vi "FPGA.vi"() -> ()   [LabVIEW 2013]
uses:
  <vilib>/Platform/TimedLoop/XDataNode/timing_clust.ctl
  <vilib>/Platform/TimedLoop/XDataNode/nitl_modes.ctl
  <vilib>/Platform/TimedLoop/XDataNode/wakeup.ctl
  <vilib>/rvi/FXPMathLib/basic elements/FxpIntAccumulator/subVIs/nifxpmath_IntAccumulator_SimConfig.ctl
  <vilib>/rvi/Emulation/niFpgaSctlEmulationGetInTimedLoop.vi
  <vilib>/rvi/Emulation/niFpgaEmulationReportErrorSimple.vi
  <vilib>/rvi/Emulation/niFpgaGetClockAttributes.vi
  <vilib>/rvi/eio/common/nirviEmuTemplateMethod_errors.vi
  <vilib>/rvi/Emulation/niFpgaCriticalErrorInLSC.vi
  <vilib>/rvi/Emulation/niFpgaProcessEmulError.vi
  <vilib>/rvi/Analysis/common/codeGenErrors/XNode/niFpgaXNodeCodeGenErrorHandle.vi
  <vilib>/rvi/FXPMathLib/basic elements/FxpIntAccumulator/simVIs/DllFxpIntAccumulator_sub.vi
  <vilib>/eio/EIONode/EIONode.xnode
  <vilib>/LabVIEW Targets/FPGA/RIO/nicrio_985x_controls.llb/CAN_IO_Frame Cluster.ctl
  <vilib>/LabVIEW Targets/FPGA/RIO/nicrio_985x_controls.llb/CAN_IO_Frame Type.ctl
  <vilib>/rvi/Analysis/measure/dc-rms/XNode/niFpgaDC-RMS.xnode
  <vilib>/Platform/TimedLoop/XDataNode/XDataNode.xnode
  <vilib>/rvi/FXPMathLib/basic elements/FxpIntAccumulator/XNode/nifxpmath_IntAccumulator.xnode
  <vilib>/rvi/FXPMathLib/FxpMul/XNode/nifxpmath_Multiplier.xnode
  <vilib>/LabVIEW Targets/FPGA/RIO/nicrio_985x_controls.llb/CAN_IO_Frame Array U32.ctl
  <vilib>/rvi/Analysis/measure/butterworth/XNode/niFpgaButterworthFilter.xnode
  <vilib>/Platform/TimedLoop/XDataNode/XDNodeRunTimeDep.lvlib
  <vilib>/rvi/FXPMathLib/sim/FxpSim.dll
panel:
  out "Licht":fxp<+/-,26,5>
  out "TorquePermitted":fxp<+/-,64,40>
  out "TD1":fxp<+/-,26,5>
  out "TD2":fxp<+/-,26,5>
  out "TD3":fxp<+/-,26,5>
  out "TD4":fxp<+/-,26,5>
  out "TD5":fxp<+/-,26,5>
  out "TD6":fxp<+/-,26,5>
  out "TD7":fxp<+/-,26,5>
  out "TD8":fxp<+/-,26,5>
  out "TD9":fxp<+/-,26,5>
  out "TD10":fxp<+/-,26,5>
  out "TD11":fxp<+/-,26,5>
  out "TD12":fxp<+/-,26,5>
  out "TD13":fxp<+/-,26,5>
  out "TD14":fxp<+/-,26,5>
  out "TD15":fxp<+/-,26,5>
  out "TD16":fxp<+/-,26,5>
  out "TD17":fxp<+/-,26,5>
  out "TD18":fxp<+/-,26,5>
  out "TD19":fxp<+/-,26,5>
  out "TD20":fxp<+/-,26,5>
  out "CurrencyDetector":fxp<+/-,26,5>
  out "Brake Detector":fxp<+/-,26,5>
  out "电池过温":bool
  out "电池过温_Sent":bool
  out "8Bytes_Received":u8[](array[numeric])
  out "ID_Received":u32
  out "1FFFFFFC":u8[](array[numeric])
  out "1FFFFFFB":u8[](array[numeric])
  out "1FFFFFFA":u8[](array[numeric])
  in  "PowerPermitted":fxp<+/-,32,8>=80.0
  in  "ErrorMonitoring?":bool
  in  "发送间隔(mSec)":u8=1 caption="Count(mSec)"
  in  "接收窗口(mSec)":u8=20 caption="Count(mSec)"
  out "0x333Byte7":u8 format="%.0b"
  out "DashSwitches":u8 format="%.0b"
  in  "CAN Input Wait?":bool
  in  "开水泵温度值":fxp<+/-,32,16>=60.0
  in  "刹车标定上限":fxp<+,32,16>=3.1199951171875
  in  "开风扇温度值":fxp<+,8,6>=45.0 format="%#_21g"
  out "AMS_fed":bool
  out "FanO?":bool
  out "PumpO?":bool
  in  "cBSPD":bool
  in  "cAMS":bool
  out "SHTD":bool
  in  "BRAKELO":bool
  in  "BUZZERO":bool
  in  "AIRNO":bool
  in  "AIRPO":bool
  in  "PREO":bool
  out "BSPD?":bool
  out "IMD?":bool
  in  "AMS":bool=TRUE
  in  "P":fxp<+,32,32>
  in  "SPD":fxp<+,32,32>
  in  "M":fxp<+,32,32>
  in  "MA":bool
  in  "BA":bool
  in  "Ready":bool
  in  "MC1TqSet_L":u8
  in  "MC1TqSet_H":u8
  in  "MC2TqSet_L":u8
  in  "MC2TqSet_H":u8
  in  "MCCmdByte":u8
  in  "BMCmdByte":u8
  out "SIG_ACC2":fxp<+/-,30,9>
  out "SIG_ACC1":fxp<+/-,30,9>
  out "SIG_BRAKE":fxp<+/-,30,9>
  out "PREC_fed":bool
  out "PREO_fed":bool
  out "50%？":bool
  out "80%？":bool
  out "SWT4?":bool
  out "SWT3?":bool
  out "Stop？":bool
  out "Start？":bool
  out "BatteryErrorRank":u8
  out "MotorErrorRank":u8
  out "AIRPO_fed":bool
  out "AIRPC_fed":bool
  out "AIRNC_fed":bool
  out "AIRNO_fed":bool
  out "BMCellVMin":fxp<+/-,32,16>
  out "BMCellVMax":fxp<+/-,32,16>
  out "BMTemMean":fxp<+/-,32,16>
  out "BMTemMax":fxp<+/-,32,16>
  out "BMTemMin":fxp<+/-,32,16>
  out "BMIdLimt":fxp<+/-,32,16>
  out "BMSStatus":u8
  out "BMSVolIs":fxp<+/-,32,16>
  out "BMSIbIs":fxp<+/-,32,16>
  out "SOCMean":fxp<+/-,32,16>
  out "LinFR":fxp<+/-,32,16>
  out "LinFL":fxp<+/-,32,16>
  out "LinRR":fxp<+/-,32,16>
  out "LinRL":fxp<+/-,32,16>
  out "W2":fxp<+,29,3>
  out "WP":fxp<+,29,3>
  out "AX":fxp<+,29,3>
  out "AY":fxp<+,29,3>
  out "AZ":fxp<+,29,3>
  out "Wr":fxp<+,29,3>
  out "ACC1":fxp<+,29,3>
  out "ACC2":fxp<+,29,3>
  out "BRK1":fxp<+,29,3>
  out "STR":fxp<+,29,3>
  out "MC2VinIs":fxp<+/-,32,16>
  out "MC2TemIs":fxp<+/-,32,16>
  out "MC2InvTemIs":fxp<+/-,32,16>
  out "MC2TqLimt":fxp<+/-,32,16>
  out "MC2Status":u8
  out "MC2SpIs":fxp<+/-,32,16>
  out "MC2TqIs":fxp<+/-,32,16>
  out "MC2ImIs":fxp<+/-,32,16>
  out "MC1VinIs":fxp<+/-,32,16>
  out "MC1TemIs":fxp<+/-,32,16>
  out "MC1InvTemIs":fxp<+/-,32,16>
  out "MC1TqLimt":fxp<+/-,32,16>
  out "MC1Status":u8
  out "MC1SpIs":fxp<+/-,32,16>
  out "MC1TqIs":fxp<+/-,32,16>
  out "MC1ImIs":fxp<+/-,32,16>
  out "PowerLimited":fxp<+/-,16,6>=1.0
  # "80kw功率限制"
  # "Digital I/O"
  # "Test Display"
  # "标定部分"
  # "CAN Sending"
  # "Analog Input"
  # "CAN Input"
  # "Motor Control"
  # "Battery Management System"
  # "Sensor Node"
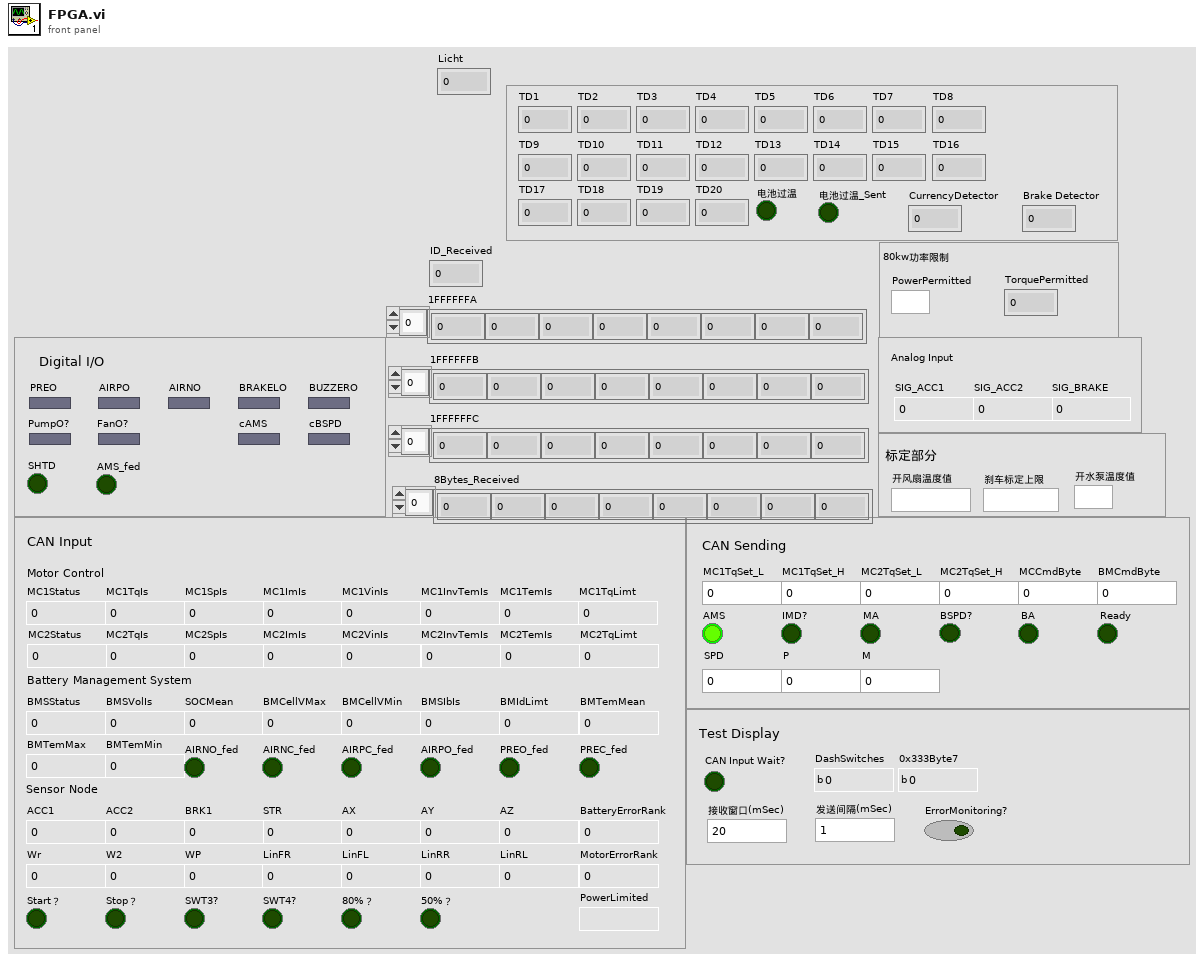
[diagram p1: front panel]
types:
  T1 = typedef "CAN_IO_Frame Cluster.ctl" = cluster{"timestamp high":u32, "timestamp low":u32, "identifier":u32, "type":T2, "info A":u8, "info B":u8, "data length":u8, "data":u8[]}
  T2 = typedef "CAN_IO_Frame Type.ctl" = enum8{"Data Frame", "Remote Frame", "(reserved)", "(reserved) ", "(reserved)  ", "(reserved)   ", "Bus Error", "Transceiver Fault"}
  T3 = typedef "XDNodeRunTimeDep.lvlib/timing_clust.ctl" = cluster{"Expected End [f-1]":u64, "Actual End [f-1]":u64, "Finished Late? [f-1]":bool, "Expected End [i-1]":u64, "Actual End [i-1]":u64, "Finished Late? [i-1]":bool, "Expected Start [i]":u64, "Actual Start [i]":u64, "Expected Start [f]":u64, "Actual Start [f]":u64, "Source Name":string, "Structure Name":string, "Period":i64, "Deadline":i64, "Offset":i64, "Start":i64, "Priority":i32, "Timeout":i32, "Mode":T4, "Wakeup Reason":T5, "Error":errorcluster, "Source Type":string, "Secondary Source Type":string, "Global End Time":u64, "Global Start Time":u64, "Frame Duration":u64, "Iteration Duration":u64, "Assigned CPU":i32, "I/O Scan Engine Mode":u32}
  T4 = typedef "XDNodeRunTimeDep.lvlib/nitl_modes.ctl" = enum32{"No Change", "Process missed periods, maintain original phase", "Discard missed periods, maintain original phase", "Process missed periods, ignore original phase", "Discard missed periods, ignore original phase"}
  T5 = typedef "XDNodeRunTimeDep.lvlib/wakeup.ctl" = enum32{"Normal", "Aborted", "Asynchronous wakeup", "Timing source error", "Timed loop error", "Timeout"}
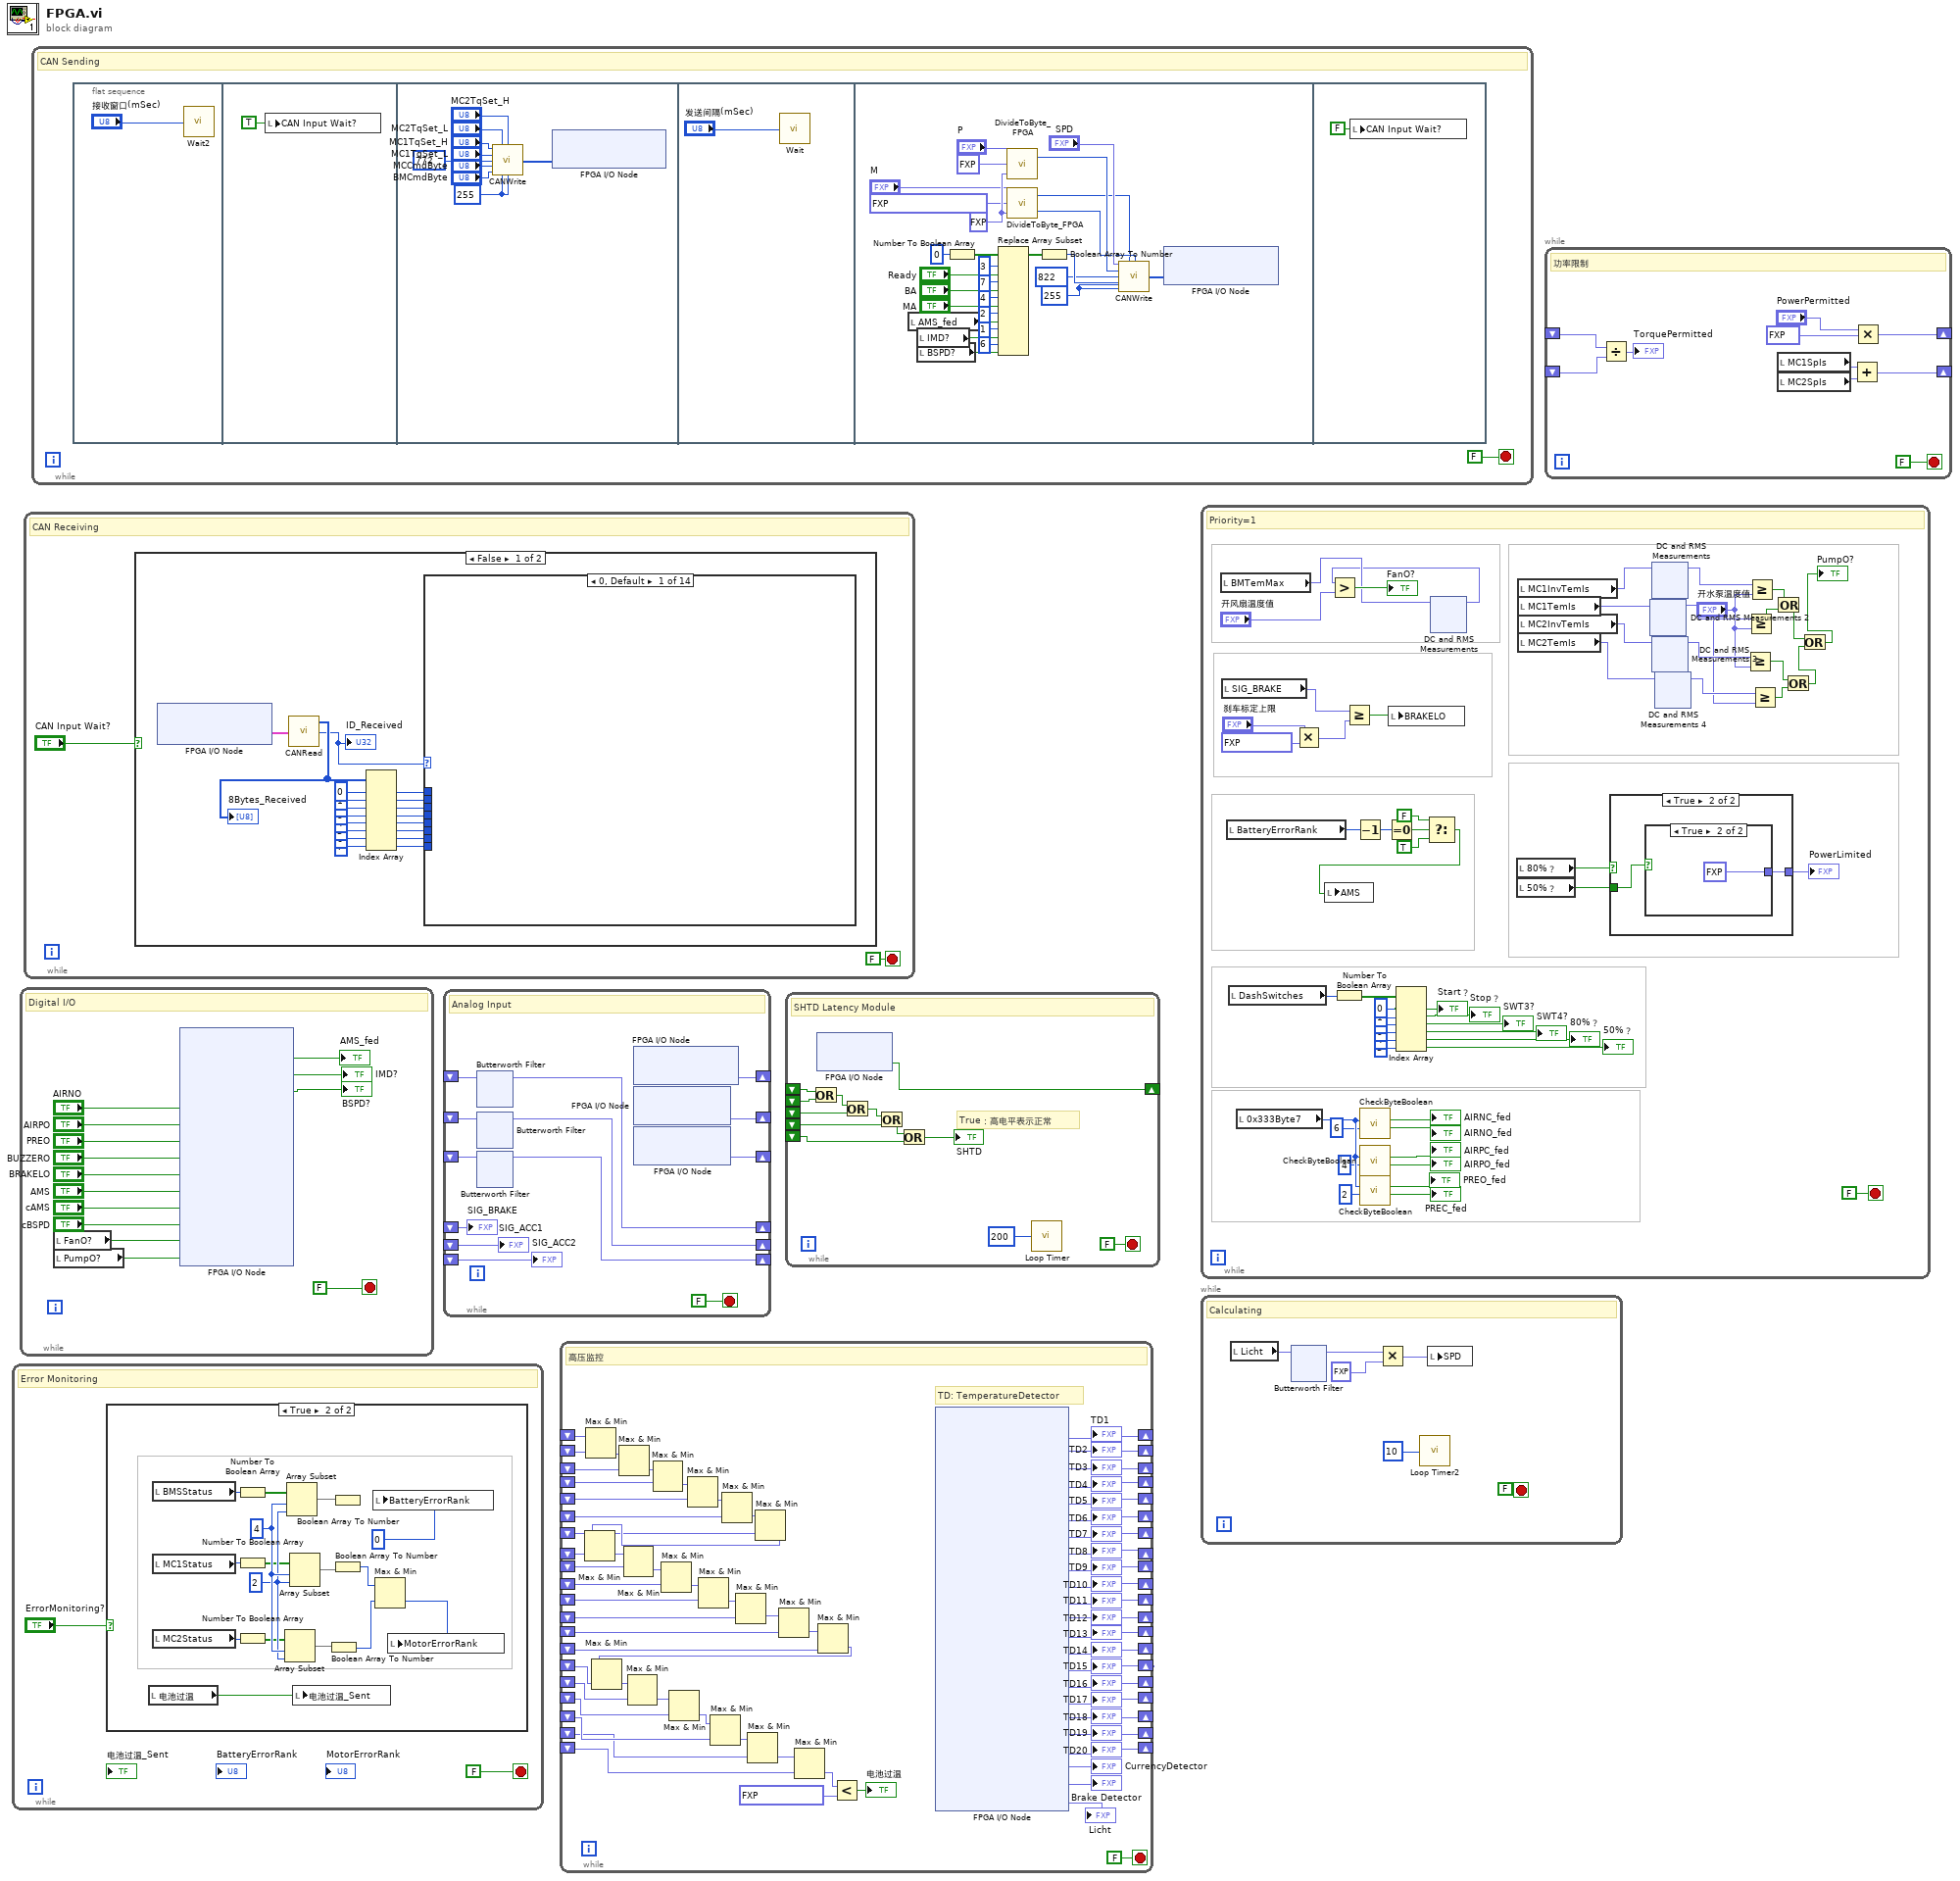
[diagram p0: block diagram]
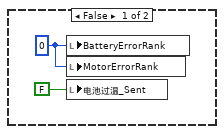
[diagram p2: hidden frame]
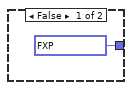
[diagram p3: hidden frame]
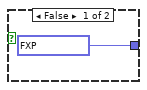
[diagram p4: hidden frame]
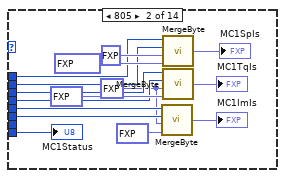
[diagram p5: hidden frame]
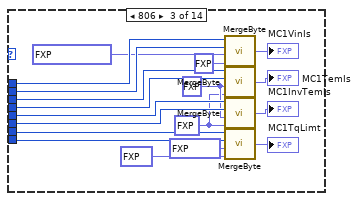
[diagram p6: hidden frame]
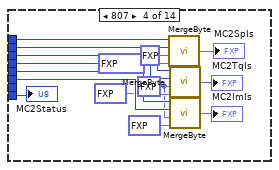
[diagram p7: hidden frame]
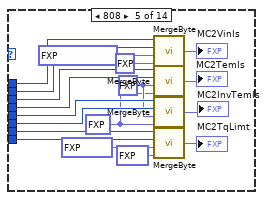
[diagram p8: hidden frame]
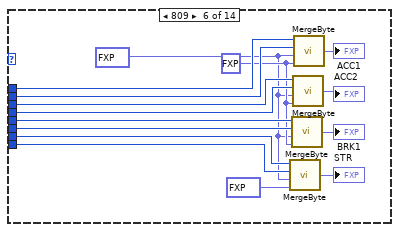
[diagram p9: hidden frame]
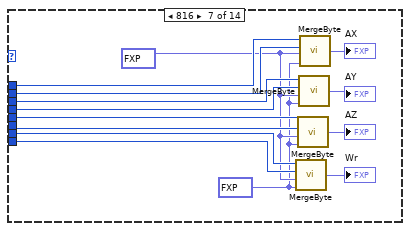
[diagram p10: hidden frame]
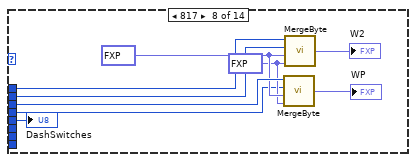
[diagram p11: hidden frame]
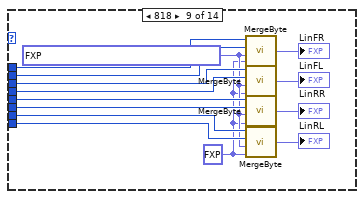
[diagram p12: hidden frame]
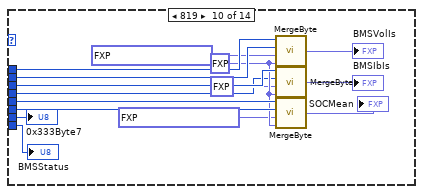
[diagram p13: hidden frame]
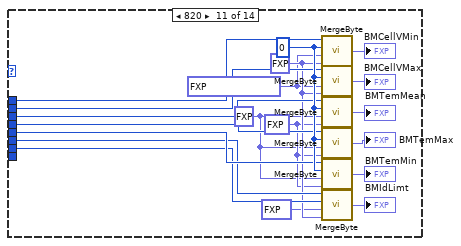
[diagram p14: hidden frame]
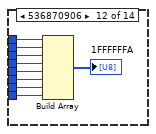
[diagram p15: hidden frame]
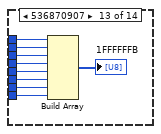
[diagram p16: hidden frame]
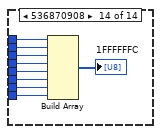
[diagram p17: hidden frame]
diagram:
  n1 = while {
    stop <- FALSE stop-if-true
    # "Error Monitoring"
    n2 = case shown="True" "ErrorMonitoring?" {
      frame False {
        w3 = u8 0 ("BatteryErrorRank")
        n3 = local write "BatteryErrorRank"(w3) -> ()
        n4 = local write "MotorErrorRank"(w3) -> ()
        n5 = local write "电池过温_Sent"(FALSE ("电池过温_Sent")) -> ()
      }
      frame True {
        w12 = 4 ("index")
        w11 = 2 ("length")
        n6 = local read "电池过温"() -> (w6:bool)
        n7 = local read "BMSStatus"() -> (w18:u8)
        n8 = local read "MC1Status"() -> (w19:u8)
        n9 = local read "MC2Status"() -> (w20:u8)
        n10 = Number To Boolean Array(number=w18) -> (Boolean array=w8:bool[])
        n11 = Number To Boolean Array(number=w19) -> (Boolean array=w9:bool[])
        n12 = Number To Boolean Array(number=w20) -> (Boolean array=w10:bool[])
        n13 = Array Subset(array=w10, index=w12, length=w11) -> (w15:bool[])
        n14 = Array Subset(array=w8, index=w12, length=w11) -> (w13:bool[])
        n15 = Array Subset(array=w9, index=w12, length=w11) -> (w14:bool[])
        n16 = local write "电池过温_Sent"(w6) -> ()
        n17 = Boolean Array To Number(Boolean array=w15) -> (number=w17:u8)
        n18 = Boolean Array To Number(Boolean array=w13) -> ()  [unwired: 1 out]
        n19 = Boolean Array To Number(Boolean array=w14) -> (number=w16:u8)
        n20 = local write "BatteryErrorRank"(u8 0 ("BatteryErrorRank")) -> ()
        n21 = Max & Min(x=w16, y=w17) -> (min(x,y)=w7:u8)  [unwired: 1 out]
        n22 = local write "MotorErrorRank"(w7) -> ()
      }
    }
  }
  n23 = while {
    stop <- FALSE stop-if-true
    # "Digital I/O"
    n24 = local read "FanO?"() -> (w22:bool)
    n25 = local read "PumpO?"() -> (w23:bool)
    n26 = xnode "FPGA I/O Node"("AIRN"="AIRNO", "AIRP"="AIRPO", "PRE"="PREO", "BUZZER"="BUZZERO", "BRAKELED"="BRAKELO", "AMS_Sent"="AMS", "controlAMS"="cAMS", "controlBSPD"="cBSPD", "FAN"=w22, "PUM2"=w23) -> ("AMS"=→"AMS_fed":bool, "IMD"=→"IMD?":bool, "BSPD"=→"BSPD?":bool)  [unwired: 13 in, 13 out]
  }
  n27 = while {
    stop <- FALSE stop-if-true
    # "CAN Receiving"
    n28 = case shown="False" "CAN Input Wait?" {
      frame False {
        n29 = xnode "FPGA I/O Node"() -> ("Mod1/CAN0"=w55:T1)  [unwired: 2 in, 2 out]
        n30 = call "CANRead.vi"("CAN Signal"=w55) -> ("8Bytes_Received"=w54:u8[], "ID_Received"=w45:u32)  [unwired: 1 in]
        "ID_Received" <- w45
        "8Bytes_Received" <- w54
        n31 = Index Array(array=w54, index #1=0 ("index"), index #2=1 ("index"), index #3=2 ("index"), index #4=3 ("index"), index #5=4 ("index"), index #6=5 ("index"), index #7=6 ("index"), index #8=7 ("index")) -> (element #1=w44:u8, element #2=w43:u8, element #3=w42:u8, element #4=w41:u8, element #5=w40:u8, element #6=w39:u8, element #7=w38:u8, element #8=w37:u8)
        n32 = case shown="0, Default" w45 {
          tunnel: w44 -> [_ w68 w88 w103 w121 w136 w146 w159 w173 w188 w206 w216 w225 w234]
          tunnel: w43 -> [_ w67 w87 w102 w120 w135 w145 w158 w172 w187 w205 w215 w224 w233]
          tunnel: w42 -> [_ w65 w86 w101 w119 w134 w144 w157 w171 w186 w204 w214 w223 w232]
          tunnel: w41 -> [_ w64 w85 w100 w118 w133 w143 w152 w170 w175 w203 w213 w222 w231]
          tunnel: w40 -> [_ w62 w84 w99 w117 w132 w142 w151 w169 w185 w202 w212 w221 w230]
          tunnel: w39 -> [_ w61 w83 w98 w116 w131 w141 _ w168 w184 w201 w211 w220 w229]
          tunnel: w38 -> [_ _ w82 _ w115 w130 w140 _ w167 w174 w200 w210 w219 w228]
          tunnel: w37 -> [_ w60 w81 w97 w114 w129 w139 _ w166 w183 _ w209 w218 w227]
          frame 0, Default {
          }
          frame 805 {
            w56 = fxp<+/-,32,16> 0.5 ("Resolution")
            n33 = call "MergeByte.vi"("Offset"=fxp<+/-,32,16> -200.0, "Resolution"=w56, "HighByte"=w61, "LowByte"=w62) -> ("Result"=→"MC1ImIs":fxp<+/-,32,16>)
            n34 = call "MergeByte.vi"("Offset"=fxp<+/-,32,16> -12000.0, "Resolution"=fxp<+/-,32,16> 1.0, "HighByte"=w67, "LowByte"=w68) -> ("Result"=→"MC1SpIs":fxp<+/-,32,16>)
            n35 = call "MergeByte.vi"("Offset"=fxp<+/-,32,16> -180.0, "Resolution"=w56, "HighByte"=w64, "LowByte"=w65) -> ("Result"=→"MC1TqIs":fxp<+/-,32,16>)
            "MC1Status" <- w60
          }
          frame 806 {
            w77 = fxp<+/-,32,16> -40.0 ("Offset")
            w78 = fxp<+/-,32,16> 1.0 ("Resolution")
            n36 = call "MergeByte.vi"("Offset"=fxp<+/-,32,16> 0.0, "Resolution"=fxp<+,8,-1> 0.349609375, "HighByte"=w87, "LowByte"=w88) -> ("Result"=→"MC1VinIs":fxp<+/-,32,16>)
            n37 = call "MergeByte.vi"("Offset"=w77, "Resolution"=w78, "HighByte"=w85, "LowByte"=w86) -> ("Result"=→"MC1TemIs":fxp<+/-,32,16>)
            n38 = call "MergeByte.vi"("Offset"=w77, "Resolution"=w78, "HighByte"=w83, "LowByte"=w84) -> ("Result"=→"MC1InvTemIs":fxp<+/-,32,16>)
            n39 = call "MergeByte.vi"("Offset"=fxp<+/-,32,16> -150.0, "Resolution"=fxp<+,5,-1> 0.40625, "HighByte"=w81, "LowByte"=w82) -> ("Result"=→"MC1TqLimt":fxp<+/-,32,16>)
          }
          frame 807 {
            w90 = fxp<+/-,32,16> 0.5 ("Resolution")
            n40 = call "MergeByte.vi"("Offset"=fxp<+/-,32,16> -12000.0, "Resolution"=fxp<+/-,32,16> 1.0, "HighByte"=w102, "LowByte"=w103) -> ("Result"=→"MC2SpIs":fxp<+/-,32,16>)
            n41 = call "MergeByte.vi"("Offset"=fxp<+/-,32,16> -150.0, "Resolution"=w90, "HighByte"=w100, "LowByte"=w101) -> ("Result"=→"MC2TqIs":fxp<+/-,32,16>)
            n42 = call "MergeByte.vi"("Offset"=fxp<+/-,32,16> -200.0, "Resolution"=w90, "HighByte"=w98, "LowByte"=w99) -> ("Result"=→"MC2ImIs":fxp<+/-,32,16>)
            "MC2Status" <- w97
          }
          frame 808 {
            w110 = fxp<+/-,32,16> -40.0 ("Offset")
            w111 = fxp<+/-,32,16> 1.0 ("Resolution")
            n43 = call "MergeByte.vi"("Offset"=fxp<+/-,32,16> 0.0, "Resolution"=fxp<+,8,-1> 0.349609375, "HighByte"=w120, "LowByte"=w121) -> ("Result"=→"MC2VinIs":fxp<+/-,32,16>)
            n44 = call "MergeByte.vi"("Offset"=w110, "Resolution"=w111, "HighByte"=w118, "LowByte"=w119) -> ("Result"=→"MC2TemIs":fxp<+/-,32,16>)
            n45 = call "MergeByte.vi"("Offset"=w110, "Resolution"=w111, "HighByte"=w116, "LowByte"=w117) -> ("Result"=→"MC2InvTemIs":fxp<+/-,32,16>)
            n46 = call "MergeByte.vi"("Offset"=fxp<+/-,32,16> -150.0, "Resolution"=fxp<+/-,32,16> 0.40625, "HighByte"=w114, "LowByte"=w115) -> ("Result"=→"MC2TqLimt":fxp<+/-,32,16>)
          }
          frame 809 {
            w124 = fxp<+/-,8,0> 0.0 ("Offset")
            w123 = fxp<+,32,30> 4095.0 ("Resolution")
            n47 = call "MergeByte.vi"("Offset"=fxp<+/-,32,16> 2048.0, "Resolution"=w123, "HighByte"=w129, "LowByte"=w130) -> ("Result"=→"STR":fxp<+/-,32,16>)
            n48 = call "MergeByte.vi"("Offset"=w124, "Resolution"=w123, "HighByte"=w131, "LowByte"=w132) -> ("Result"=→"BRK1":fxp<+/-,32,16>)
            n49 = call "MergeByte.vi"("Offset"=w124, "Resolution"=w123, "HighByte"=w133, "LowByte"=w134) -> ("Result"=→"ACC2":fxp<+/-,32,16>)
            n50 = call "MergeByte.vi"("Offset"=w124, "Resolution"=w123, "HighByte"=w135, "LowByte"=w136) -> ("Result"=→"ACC1":fxp<+/-,32,16>)
          }
          frame 816 {
            w137 = fxp<+/-,32,30> 2048.0 ("Offset")
            w138 = fxp<+,32,30> 4095.0 ("Resolution")
            n51 = call "MergeByte.vi"("Offset"=w137, "Resolution"=w138, "HighByte"=w139, "LowByte"=w140) -> ("Result"=→"Wr":fxp<+/-,32,16>)
            n52 = call "MergeByte.vi"("Offset"=w137, "Resolution"=w138, "HighByte"=w141, "LowByte"=w142) -> ("Result"=→"AZ":fxp<+/-,32,16>)
            n53 = call "MergeByte.vi"("Offset"=w137, "Resolution"=w138, "HighByte"=w143, "LowByte"=w144) -> ("Result"=→"AY":fxp<+/-,32,16>)
            n54 = call "MergeByte.vi"("Offset"=w137, "Resolution"=w138, "HighByte"=w145, "LowByte"=w146) -> ("Result"=→"AX":fxp<+/-,32,16>)
          }
          frame 817 {
            w153 = fxp<+/-,32,30> 2048.0 ("Offset")
            w156 = fxp<+,32,30> 4095.0 ("Resolution")
            n55 = call "MergeByte.vi"("Offset"=w153, "Resolution"=w156, "HighByte"=w152, "LowByte"=w157) -> ("Result"=→"WP":fxp<+/-,32,16>)
            n56 = call "MergeByte.vi"("Offset"=w153, "Resolution"=w156, "HighByte"=w158, "LowByte"=w159) -> ("Result"=→"W2":fxp<+/-,32,16>)
            "DashSwitches" <- w151
          }
          frame 818 {
            w164 = fxp<+/-,32,16> 0.0 ("Offset")
            w165 = fxp<+,24,-2> 0.0016113370656967163 ("Resolution")
            n57 = call "MergeByte.vi"("Offset"=w164, "Resolution"=w165, "HighByte"=w172, "LowByte"=w173) -> ("Result"=→"LinFR":fxp<+/-,32,16>)
            n58 = call "MergeByte.vi"("Offset"=w164, "Resolution"=w165, "HighByte"=w170, "LowByte"=w171) -> ("Result"=→"LinFL":fxp<+/-,32,16>)
            n59 = call "MergeByte.vi"("Offset"=w164, "Resolution"=w165, "HighByte"=w168, "LowByte"=w169) -> ("Result"=→"LinRR":fxp<+/-,32,16>)
            n60 = call "MergeByte.vi"("Offset"=w164, "Resolution"=w165, "HighByte"=w166, "LowByte"=w167) -> ("Result"=→"LinRL":fxp<+/-,32,16>)
          }
          frame 819 {
            w179 = fxp<+/-,32,16> 0.0 ("Offset")
            n61 = call "MergeByte.vi"("Offset"=w179, "Resolution"=fxp<+/-,32,16> 0.100006103515625, "HighByte"=w187, "LowByte"=w188) -> ("Result"=→"BMSVolIs":fxp<+/-,32,16>)
            n62 = call "MergeByte.vi"("Offset"=w179, "Resolution"=fxp<+/-,32,16> 0.5, "HighByte"=w175, "LowByte"=w186) -> ("Result"=→"BMSIbIs":fxp<+/-,32,16>)
            n63 = call "MergeByte.vi"("Offset"=w179, "Resolution"=fxp<+/-,32,16> 0.149993896484375, "HighByte"=w184, "LowByte"=w185) -> ("Result"=→"SOCMean":fxp<+/-,32,16>)
            "BMSStatus" <- w183
            "0x333Byte7" <- w174
          }
          frame 820 {
            w196 = fxp<+/-,32,16> 1.0 ("Resolution")
            w197 = fxp<+,6,-5> 0.02001953125 ("Resolution")
            w198 = fxp<+/-,32,16> -40.0 ("Offset")
            w199 = fxp<+/-,32,16> 0.0 ("Offset")
            w207 = u8 0 ("HighByte")
            n64 = call "MergeByte.vi"("Offset"=w199, "Resolution"=w197, "HighByte"=w207, "LowByte"=w206) -> ("Result"=→"BMCellVMin":fxp<+/-,32,16>)
            n65 = call "MergeByte.vi"("Offset"=w199, "Resolution"=w197, "HighByte"=w207, "LowByte"=w205) -> ("Result"=→"BMCellVMax":fxp<+/-,32,16>)
            n66 = call "MergeByte.vi"("Offset"=w198, "Resolution"=w196, "HighByte"=w207, "LowByte"=w204) -> ("Result"=→"BMTemMean":fxp<+/-,32,16>)
            n67 = call "MergeByte.vi"("Offset"=w198, "Resolution"=w196, "HighByte"=w207, "LowByte"=w203) -> ("Result"=→"BMTemMax":fxp<+/-,32,16>)
            n68 = call "MergeByte.vi"("Offset"=w198, "Resolution"=w196, "HighByte"=w207, "LowByte"=w202) -> ("Result"=→"BMTemMin":fxp<+/-,32,16>)
            n69 = call "MergeByte.vi"("Offset"=w199, "Resolution"=fxp<+/-,32,16> 0.25, "HighByte"=w200, "LowByte"=w201) -> ("Result"=→"BMIdLimt":fxp<+/-,32,16>)
          }
          frame 536870906 {
            n70 = Build Array(w216, w215, w214, w213, w212, w211, w210, w209) -> (→"1FFFFFFA":u8[])
          }
          frame 536870907 {
            n71 = Build Array(w225, w224, w223, w222, w221, w220, w219, w218) -> (→"1FFFFFFB":u8[])
          }
          frame 536870908 {
            n72 = Build Array(w234, w233, w232, w231, w230, w229, w228, w227) -> (→"1FFFFFFC":u8[])
          }
        }
      }
      frame True {
      }
    }
  }
  n73 = while {
    stop <- FALSE stop-if-true
    # "CAN Sending"
    n74 = flat-sequence {
      frame #0 {
        n75 = call "Wait2"("Count(mSec)"="接收窗口(mSec)") -> ()  [unwired: 1 out]
      }
      frame #1 {
        n76 = local write "CAN Input Wait?"(TRUE ("CAN Input Wait?")) -> ()
      }
      frame #2 {
        w238 = u8 255
        n77 = call "CANWrite.vi"("Data1"="MC1TqSet_H", "Data2"="MC2TqSet_L", "Data3"="MC2TqSet_H", "Data0"="MC1TqSet_L", "ID_ToSend"=u32 772, "Data4"="MCCmdByte", "Data5"="BMCmdByte", "Data6"=w238, "Data7"=w238) -> ("Frame"=w240:u32[])  [unwired: 6 in]
        n78 = xnode "FPGA I/O Node"("Mod1/CAN0"=w240) -> ()  [unwired: 1 in, 1 out]
      }
      frame #3 {
        n79 = call "Wait"("Count(mSec)"="发送间隔(mSec)") -> ()  [unwired: 1 out]
      }
      frame #4 {
        w272 = fxp<+/-,64,32> 0.0 ("Offset")
        w263 = u8 255 ("Data7")
        n80 = local read "AMS_fed"() -> (w273:bool)
        n81 = local read "IMD?"() -> (w274:bool)
        n82 = local read "BSPD?"() -> (w275:bool)
        n83 = Number To Boolean Array(number=u8 0) -> (Boolean array=w251:bool[])
        n84 = Replace Array Subset(array=w251, new element #1="Ready", index #1=u8 3 ("index"), new element #2="BA", index #2=u8 7 ("index"), new element #3="MA", index #3=u8 4 ("index"), new element #4=w273, index #4=u8 2 ("index"), new element #5=w274, index #5=u8 1 ("index"), new element #6=w275, index #6=u8 6 ("index")) -> (w252:bool[])
        n85 = call "DivideToByte_FPGA.vi"("Offset"=w272, "Resolution"=fxp<+/-,64,32> 0.5, "Value"="P") -> ("LowByte"=w269:u8)  [unwired: 1 out]
        n86 = call "DivideToByte_FPGA.vi"("Offset"=w272, "Resolution"=fxp<+/-,32,16> 0.100006103515625, "Value"="M") -> ("HighByte"=w265:u8, "LowByte"=w264:u8)
        n87 = Boolean Array To Number(Boolean array=w252) -> (number=w262:u8)
        n88 = call "CANWrite.vi"("Data1"="SPD", "Data2"=w264, "Data3"=w265, "Data0"=w269, "ID_ToSend"=u32 822, "Data4"=w262, "Data5"=w263, "Data6"=w263, "Data7"=w263) -> ("Frame"=w249:u32[])  [unwired: 6 in]
        n89 = xnode "FPGA I/O Node"("Mod1/CAN0"=w249) -> ()  [unwired: 1 in, 1 out]
      }
      frame #5 {
        n90 = local write "CAN Input Wait?"(FALSE ("CAN Input Wait?")) -> ()
      }
    }
  }
  n91 = while {
    shift-right: [w288] -> _
    shift-left: _ -> [w287]
    shift-right: [w286] -> _
    shift-left: _ -> [w285]
    shift-right: [w284] -> _
    shift-left: _ -> [w283]
    shift-right: [w282] -> _
    shift-left: _ -> [w279]
    shift-right: [w281] -> _
    shift-left: _ -> [w278]
    shift-right: [w280] -> _
    shift-left: _ -> [w277]
    stop <- FALSE stop-if-true
    # "Analog Input"
    n92 = xnode "Butterworth Filter"("input data"=w287) -> ("output data"=w282:fxp<+/-,30,9>)  [unwired: 2 in]
    n93 = xnode "Butterworth Filter"("input data"=w285) -> ("output data"=w281:fxp<+/-,30,9>)  [unwired: 2 in]
    n94 = xnode "Butterworth Filter"("input data"=w283) -> ("output data"=w280:fxp<+/-,30,9>)  [unwired: 2 in]
    n95 = xnode "FPGA I/O Node"() -> ("SIG_BRAKE"=w288:fxp<+/-,26,5>)  [unwired: 1 in, 1 out]
    n96 = xnode "FPGA I/O Node"() -> ("SIG_ACC1"=w286:fxp<+/-,26,5>)  [unwired: 1 in, 1 out]
    n97 = xnode "FPGA I/O Node"() -> ("SIG_ACC2"=w284:fxp<+/-,26,5>)  [unwired: 1 in, 1 out]
    "SIG_BRAKE" <- w279
    "SIG_ACC1" <- w278
    "SIG_ACC2" <- w277
  }
  n98 = while {
    shift-right: [w375] -> _
    shift-left: _ -> [w355]
    shift-right: [w374] -> _
    shift-left: _ -> [w354]
    shift-right: [w373] -> _
    shift-left: _ -> [w352]
    shift-right: [w372] -> _
    shift-left: _ -> [w339]
    shift-right: [w371] -> _
    shift-left: _ -> [w338]
    shift-right: [w370] -> _
    shift-left: _ -> [w337]
    shift-right: [w369] -> _
    shift-left: _ -> [w336]
    shift-right: [w368] -> _
    shift-left: _ -> [w335]
    shift-right: [w367] -> _
    shift-left: _ -> [w334]
    shift-right: [w366] -> _
    shift-left: _ -> [w333]
    shift-right: [w365] -> _
    shift-left: _ -> [w332]
    shift-right: [w364] -> _
    shift-left: _ -> [w331]
    shift-right: [w363] -> _
    shift-left: _ -> [w330]
    shift-right: [w362] -> _
    shift-left: _ -> [w328]
    shift-right: [w361] -> _
    shift-left: _ -> [w325]
    shift-right: [w360] -> _
    shift-left: _ -> [w324]
    shift-right: [w359] -> _
    shift-left: _ -> [w322]
    shift-right: [w358] -> _
    shift-left: _ -> [w320]
    shift-right: [w357] -> _
    shift-left: _ -> [w318]
    shift-right: [w356] -> _
    shift-left: _ -> [w316]
    stop <- FALSE stop-if-true
    # "TD: TemperatureDetector"
    # "高压监控"
    n99 = Max & Min(x=w355, y=w354) -> (min(x,y)=w353:fxp<+/-,26,5>)  [unwired: 1 out]
    n100 = Max & Min(x=w353, y=w352) -> (min(x,y)=w340:fxp<+/-,26,5>)  [unwired: 1 out]
    n101 = Max & Min(x=w340, y=w339) -> (min(x,y)=w351:fxp<+/-,26,5>)  [unwired: 1 out]
    n102 = Max & Min(x=w351, y=w338) -> (min(x,y)=w350:fxp<+/-,26,5>)  [unwired: 1 out]
    n103 = Max & Min(x=w350, y=w337) -> (min(x,y)=w349:fxp<+/-,26,5>)  [unwired: 1 out]
    n104 = Max & Min(x=w349, y=w336) -> (min(x,y)=w348:fxp<+/-,26,5>)  [unwired: 1 out]
    n105 = Max & Min(x=w348, y=w335) -> (min(x,y)=w347:fxp<+/-,26,5>)  [unwired: 1 out]
    n106 = Max & Min(x=w347, y=w334) -> (min(x,y)=w346:fxp<+/-,26,5>)  [unwired: 1 out]
    n107 = Max & Min(x=w346, y=w333) -> (min(x,y)=w345:fxp<+/-,26,5>)  [unwired: 1 out]
    n108 = Max & Min(x=w345, y=w332) -> (min(x,y)=w344:fxp<+/-,26,5>)  [unwired: 1 out]
    n109 = Max & Min(x=w344, y=w331) -> (min(x,y)=w343:fxp<+/-,26,5>)  [unwired: 1 out]
    n110 = Max & Min(x=w343, y=w330) -> (min(x,y)=w329:fxp<+/-,26,5>)  [unwired: 1 out]
    n111 = Max & Min(x=w329, y=w328) -> (min(x,y)=w327:fxp<+/-,26,5>)  [unwired: 1 out]
    n112 = Max & Min(x=w327, y=w325) -> (min(x,y)=w326:fxp<+/-,26,5>)  [unwired: 1 out]
    n113 = Max & Min(x=w326, y=w324) -> (min(x,y)=w323:fxp<+/-,26,5>)  [unwired: 1 out]
    n114 = Max & Min(x=w323, y=w322) -> (min(x,y)=w321:fxp<+/-,26,5>)  [unwired: 1 out]
    n115 = Max & Min(x=w321, y=w320) -> (min(x,y)=w319:fxp<+/-,26,5>)  [unwired: 1 out]
    n116 = Max & Min(x=w319, y=w318) -> (min(x,y)=w317:fxp<+/-,26,5>)  [unwired: 1 out]
    n117 = Max & Min(x=w317, y=w316) -> (min(x,y)=w315:fxp<+/-,26,5>)  [unwired: 1 out]
    n118 = Less?(x=w315, y=fxp<+/-,16,2> 0.9912109375) -> (x < y?=→"电池过温":bool)
    n119 = xnode "FPGA I/O Node"() -> ("TD1"=w375:fxp<+/-,26,5>, "TD2"=w374:fxp<+/-,26,5>, "TD3"=w373:fxp<+/-,26,5>, "TD4"=w372:fxp<+/-,26,5>, "TD5"=w371:fxp<+/-,26,5>, "TD6"=w370:fxp<+/-,26,5>, "TD7"=w369:fxp<+/-,26,5>, "TD8"=w368:fxp<+/-,26,5>, "TD9"=w367:fxp<+/-,26,5>, "TD10"=w366:fxp<+/-,26,5>, "TD11"=w365:fxp<+/-,26,5>, "TD12"=w364:fxp<+/-,26,5>, "TD13"=w363:fxp<+/-,26,5>, "TD14"=w362:fxp<+/-,26,5>, "TD15"=w361:fxp<+/-,26,5>, "TD16"=w360:fxp<+/-,26,5>, "TD17"=w359:fxp<+/-,26,5>, "TD18"=w358:fxp<+/-,26,5>, "TD19"=w357:fxp<+/-,26,5>, "TD20"=w356:fxp<+/-,26,5>, "CurrentDetector"=→"CurrencyDetector":fxp<+/-,26,5>, "BrakeDetector"=→"Brake Detector":fxp<+/-,26,5>, "Licht"=→"Licht":fxp<+/-,26,5>)  [unwired: 23 in, 23 out]
    "TD1" <- w375
    "TD2" <- w374
    "TD3" <- w373
    "TD4" <- w372
    "TD5" <- w371
    "TD6" <- w370
    "TD7" <- w369
    "TD8" <- w368
    "TD9" <- w367
    "TD10" <- w366
    "TD11" <- w365
    "TD12" <- w364
    "TD13" <- w363
    "TD14" <- w362
    "TD15" <- w361
    "TD16" <- w360
    "TD17" <- w359
    "TD18" <- w358
    "TD19" <- w357
    "TD20" <- w356
  }
  n120 = while {
    shift-right: [w389] -> _
    shift-left: _ -> [w388]
    shift-left: _ -> [w387]
    shift-left: _ -> [w385]
    shift-left: _ -> [w383]
    shift-left: _ -> [w382]
    stop <- FALSE stop-if-true
    # "True：高电平表示正常"
    # "SHTD Latency Module"
    n121 = Or(x=w388, y=w387) -> (x .or. y?=w386:bool)
    n122 = xnode "FPGA I/O Node"() -> ("SHTD"=w389:bool)  [unwired: 1 in, 1 out]
    n123 = Or(x=w386, y=w385) -> (x .or. y?=w384:bool)
    n124 = Or(x=w384, y=w383) -> (x .or. y?=w381:bool)
    n125 = Or(x=w381, y=w382) -> (x .or. y?=→"SHTD":bool)
    n126 = call "Loop Timer"("Count(mSec)"=u8 200) -> ()  [unwired: 1 out]
  }
  n127 = while {
    stop <- FALSE stop-if-true
    # "Priority=1"
    n128 = local read "BMTemMax"() -> (w399:fxp<+/-,32,16>)
    n129 = local read "SIG_BRAKE"() -> (w419:fxp<+/-,30,9>)
    n130 = local read "BatteryErrorRank"() -> (w397:u8)
    n131 = local read "DashSwitches"() -> (w431:u8)
    n132 = local read "0x333Byte7"() -> (w430:u8)
    n133 = Multiply(x="刹车标定上限", y=fxp<+,8,-1> 0.44921875) -> (x*y=w416:fxp<+,40,15>)
    n134 = Number To Boolean Array(number=w431) -> (Boolean array=w432:bool[])
    n135 = Greater Or Equal?(x=w419, y=w416) -> (x >= y?=w415:bool)
    n136 = Decrement(x=w397) -> (x-1=w396:u8)
    n137 = call "CheckByteBoolean.vi"("SingleByte"=w430, "StartIndex"=u8 6) -> ("=10？"=→"AIRNC_fed":bool, "=01？"=→"AIRNO_fed":bool)  [unwired: 6 in]
    n138 = call "CheckByteBoolean.vi"("SingleByte"=w430, "StartIndex"=u8 4) -> ("=10？"=→"AIRPC_fed":bool, "=01？"=→"AIRPO_fed":bool)  [unwired: 6 in]
    n139 = call "CheckByteBoolean.vi"("SingleByte"=w430, "StartIndex"=u8 2) -> ("=10？"=→"PREO_fed":bool, "=01？"=→"PREC_fed":bool)  [unwired: 6 in]
    n140 = Equal To 0?(x=w396) -> (x = 0?=w395:bool)
    n141 = local write "BRAKELO"(w415) -> ()
    n142 = Index Array(array=w432, index #1=0 ("index"), index #2=1 ("index"), index #3=2 ("index"), index #4=3 ("index"), index #5=4 ("index"), index #6=5 ("index")) -> (element #1=→"Start？":bool, element #2=→"Stop？":bool, element #3=→"SWT3?":bool, element #4=→"SWT4?":bool, element #5=→"80%？":bool, element #6=→"50%？":bool)
    n143 = Select(t=FALSE, s=w395, f=TRUE) -> (s? t:f=w392:bool)
    n144 = local write "AMS"(w392) -> ()
    n145 = xnode "DC and RMS Measurements"("input data"=w399) -> ("DC"=w398:fxp<+/-,32,16>)  [unwired: 1 in, 1 out]
    n146 = Greater?(x=w398, y="开风扇温度值") -> (0:→"FanO?":bool)
    n147 = local read "80%？"() -> (w446:bool)
    n148 = local read "50%？"() -> (w445:bool)
    n149 = local read "MC1InvTemIs"() -> (w414:fxp<+/-,32,16>)
    n150 = local read "MC1TemIs"() -> (w413:fxp<+/-,32,16>)
    n151 = local read "MC2InvTemIs"() -> (w412:fxp<+/-,32,16>)
    n152 = local read "MC2TemIs"() -> (w411:fxp<+/-,32,16>)
    n153 = case shown="True" w446 {
      tunnel: w445 -> [_ w852]
      tunnel: [fxp<+,8,0> 0.99609375 ("功率限制百分比") w851] -> w447
      frame False {
      }
      frame True {
        n154 = case shown="True" w852 {
          tunnel: [fxp<+,8,0> 0.80078125 ("功率限制百分比") fxp<+,8,0> 0.5 ("功率限制百分比")] -> w851
          frame False {
          }
          frame True {
          }
        }
      }
    }
    "PowerLimited" <- w447
    n155 = xnode ("DC and RMS Measurements 2")("input data"=w413) -> ("DC"=w409:fxp<+/-,32,16>)  [unwired: 1 in, 1 out]
    n156 = xnode ("DC and RMS Measurements")("input data"=w414) -> ("DC"=w410:fxp<+/-,32,16>)  [unwired: 1 in, 1 out]
    n157 = xnode ("DC and RMS Measurements 3")("input data"=w412) -> ("DC"=w408:fxp<+/-,32,16>)  [unwired: 1 in, 1 out]
    n158 = xnode ("DC and RMS Measurements 4")("input data"=w411) -> ("DC"=w407:fxp<+/-,32,16>)  [unwired: 1 in, 1 out]
    n159 = Greater Or Equal?(x=w408, y="开水泵温度值") -> (x >= y?=w403:bool)
    n160 = Greater Or Equal?(x=w409, y="开水泵温度值") -> (x >= y?=w405:bool)
    n161 = Greater Or Equal?(x=w410, y="开水泵温度值") -> (x >= y?=w406:bool)
    n162 = Greater Or Equal?(x=w407, y="开水泵温度值") -> (x >= y?=w404:bool)
    n163 = Or(x=w406, y=w405) -> (x .or. y?=w402:bool)
    n164 = Or(x=w403, y=w404) -> (x .or. y?=w401:bool)
    n165 = Or(x=w402, y=w401) -> (x .or. y?=→"PumpO?":bool)
  }
  n166 = while {
    stop <- FALSE stop-if-true
    # "Calculating"
    n167 = local read "Licht"() -> (w859:fxp<+/-,26,5>)
    n168 = xnode "Butterworth Filter"("input data"=w859) -> ("output data"=w858:fxp<+/-,30,9>)  [unwired: 2 in]
    n169 = Multiply(x=w858, y=fxp<+/-,30,9> 25.0) -> (x*y=w856:fxp<+/-,60,18>)
    n170 = call "Loop Timer2"("Count(mSec)"=u8 10) -> ()  [unwired: 1 out]
    n171 = local write "SPD"(w856) -> ()
  }
  n172 = while {
    shift-right: [w872] -> _
    shift-left: _ -> [w870]
    shift-right: [w871] -> _
    shift-left: _ -> [w869]
    stop <- FALSE stop-if-true
    # "功率限制"
    n173 = Divide(x=w870, y=w869) -> (x/y=→"TorquePermitted":fxp<+/-,64,40>)
    n174 = local read "MC1SpIs"() -> (w874:fxp<+/-,32,16>)
    n175 = local read "MC2SpIs"() -> (w875:fxp<+/-,32,16>)
    n176 = Add(x=w874, y=w875) -> (x+y=w871:fxp<+/-,33,17>)
    n177 = Multiply(x="PowerPermitted", y=fxp<+,16,16> 9550.0) -> (x*y=w872:fxp<+/-,48,24>)
  }
